vi "Sample Transfer Get Purge Times.vi"(8 "error in (no error)":errorcluster, 11 "cRIO-CO2 in":refnum<class "cRIO-CO2.lvclass">) -> (0 "error out":errorcluster, 1 "Purge Time (sec)":dbl, 2 "Purge Capillary Time (sec)":dbl, 3 "cRIO-CO2 out":refnum<class "cRIO-CO2.lvclass">)   [LabVIEW 2015, in "cRIO-Carbondioxide.lvlib" / "cRIO-CO2.lvlib" / "cRIO-CO2.lvclass"]
uses:
  cRIO-CO2.lvclass
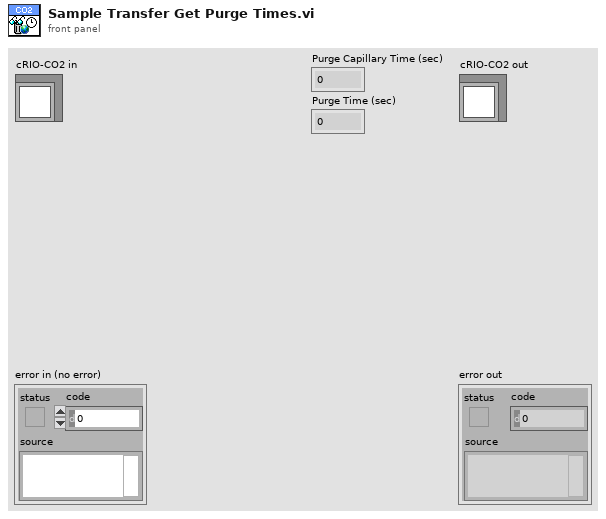
[diagram p1: front panel]
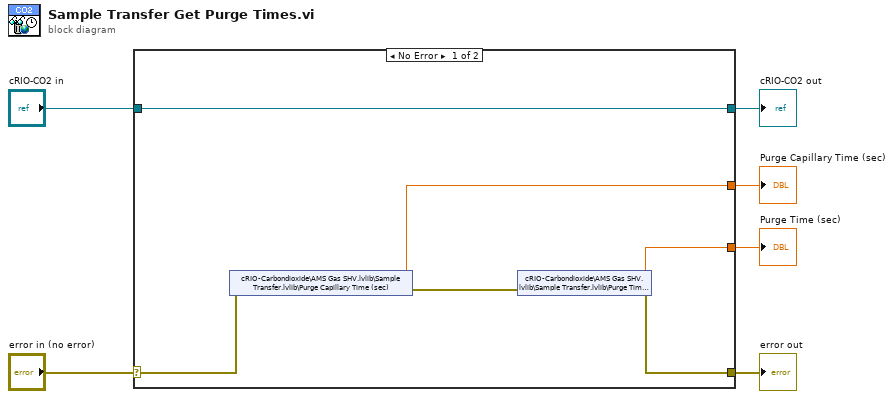
[diagram p0: block diagram]
diagram:
  n1 = case shown="No Error" "error in (no error)" {
    selector: "error in (no error)" -> [w10 w14]
    tunnel: [w9 w14] -> w5
    tunnel: [w12 w13] -> w3
    tunnel: "cRIO-CO2 in" -> [w12 w13]
    tunnel: [w8 _] -> w2
    tunnel: [w7 _] -> w1
    frame No Error {
      n2 = shared-variable "cRIO-Carbondioxide\\AMS Gas SHV.lvlib\\Sample Transfer.lvlib\\Purge Capillary Time (sec)"(error in=w10) -> (w8:dbl, error out=w11:errorcluster)
      n3 = shared-variable "cRIO-Carbondioxide\\AMS Gas SHV.lvlib\\Sample Transfer.lvlib\\Purge Time (sec)"(error in=w11) -> (w7:dbl, error out=w9:errorcluster)
    }
    frame Error {
    }
  }
  "error out" <- w5
  "cRIO-CO2 out" <- w3
  "Purge Capillary Time (sec)" <- w2
  "Purge Time (sec)" <- w1
